vi "Read Encoders 1.vi"(8 "error in (no error)":errorcluster, 9 "No samples":u32=1000, 11 "task in":i32) -> (0 "error out":errorcluster, 3 "task out":i32)   [LabVIEW 2023]
uses:
  <userlib>/DAQNavi Polymorphic VI/read/DAQNavi Read (Digital 2D U8 NChan NSamp).vi
panel:
  out "data":u8[][](array[numeric])
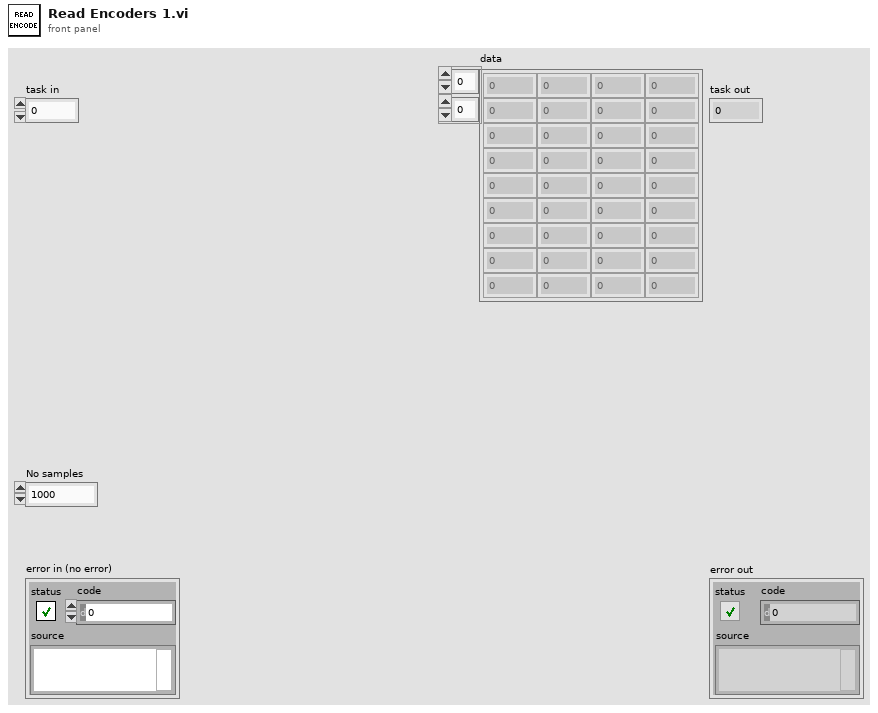
[diagram p1: front panel]
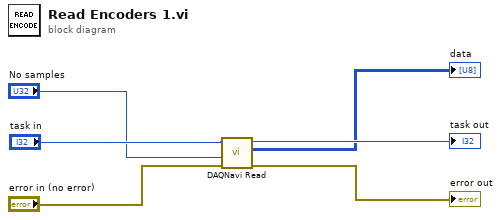
[diagram p0: block diagram]
diagram:
  n1 = call-poly <userlib>:"DAQNavi Read.vi"("error in (no error)"="error in (no error)", "number of samples per channel to read"="No samples", "task in"="task in") -> ("error out"=→"error out":errorcluster, "data"=→"data":u8[][], "task out"=→"task out":i32)  [unwired: 1 in, 5 out]
